vi "ROSTerminal.vi"() -> ()   [LabVIEW 2012]
doc: "Provides a space to debug any errors in code by:\n-allowing for testing connection to master\n-showing open nodes\n-linking to a website for viewing what is passed back and forth on a topic\n-linking to a website for the master to view what is passed back and forth\n-showing open logs\n-providing IP for you and Master"
uses:
  <userlib>/ROS for LabVIEW Software/ROS/Code/SubVIs/_ROSControl.ctl
  <userlib>/ROS for LabVIEW Software/ROS/Code/SubVIs/_ROSDirection.ctl
  <userlib>/ROS for LabVIEW Software/ROS/Code/_ROSDefinition.vi
  <vilib>/Platform/browser.llb/Open URL in Default Browser (string).vi
panel:
  in  "CloseServer":bool
  out "Queue Contents":string[](array[string])
  in  "ClearAllLogs":bool
  in  "CloseServers":bool
  in  "LabVIEW Servers":i32(listbox)
  in  "ClearOldLogs":bool
  in  "Web Logs":i32(listbox)
  in  "OpenNodes":bool
  in  "MasterWeb":bool
  in  "MyWeb":bool
  in  "UDP":bool
  out "My IP":string="http://192.168.1.8"
  in  "Done":bool
  out "Live":bool
  in  "Test":bool
  in  "Current Master":string="192.168.1.110:11311"
  # "Displays queue size and contents. Double click for\nmore information on a particular server."
  # "Show commands sent over TCP. \nDouble click to open a web page."
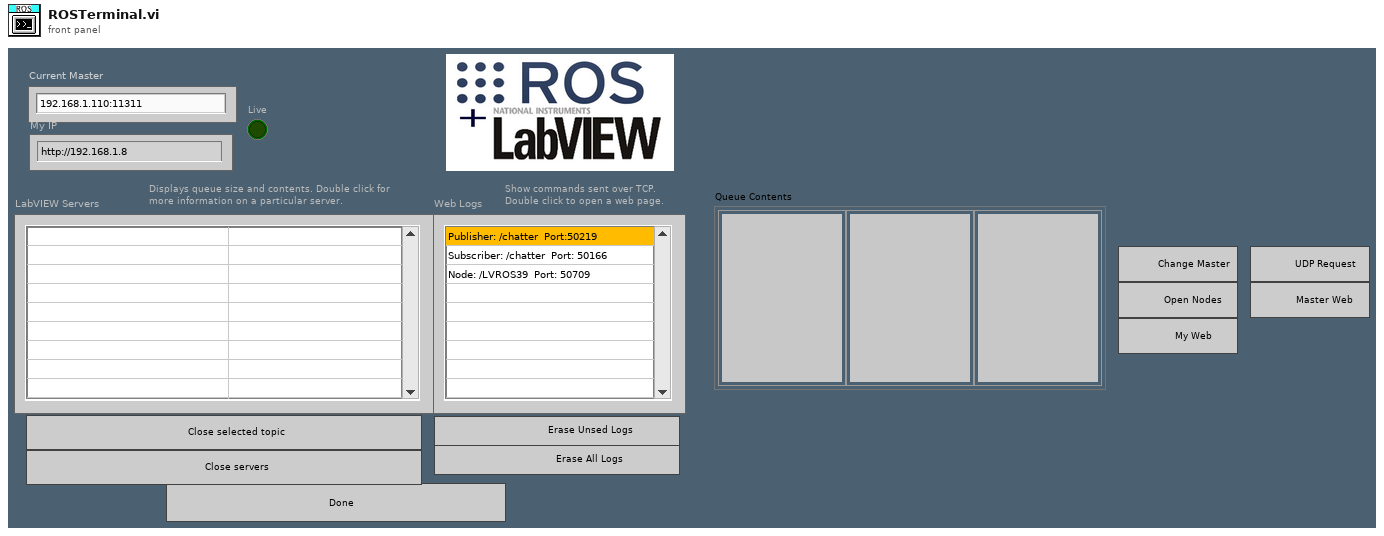
[diagram p1: front panel]
types:
  T1 = enum8{"Enabled", "Disabled", "Disabled and Grayed Out"}
  T2 = typedef "_ROSControl.ctl" = cluster{"topic port":u16, "Node":string, "topic":string, "type":string, "node port":u16, "error ":errorcluster, "Direction":T3, "Update (ms)":u16, "FIFO size":u16}
  T3 = typedef "_ROSDirection.ctl" = enum16{"Node", "Publisher", "Subscriber", "ServiceClient", "ServiceProvider"}
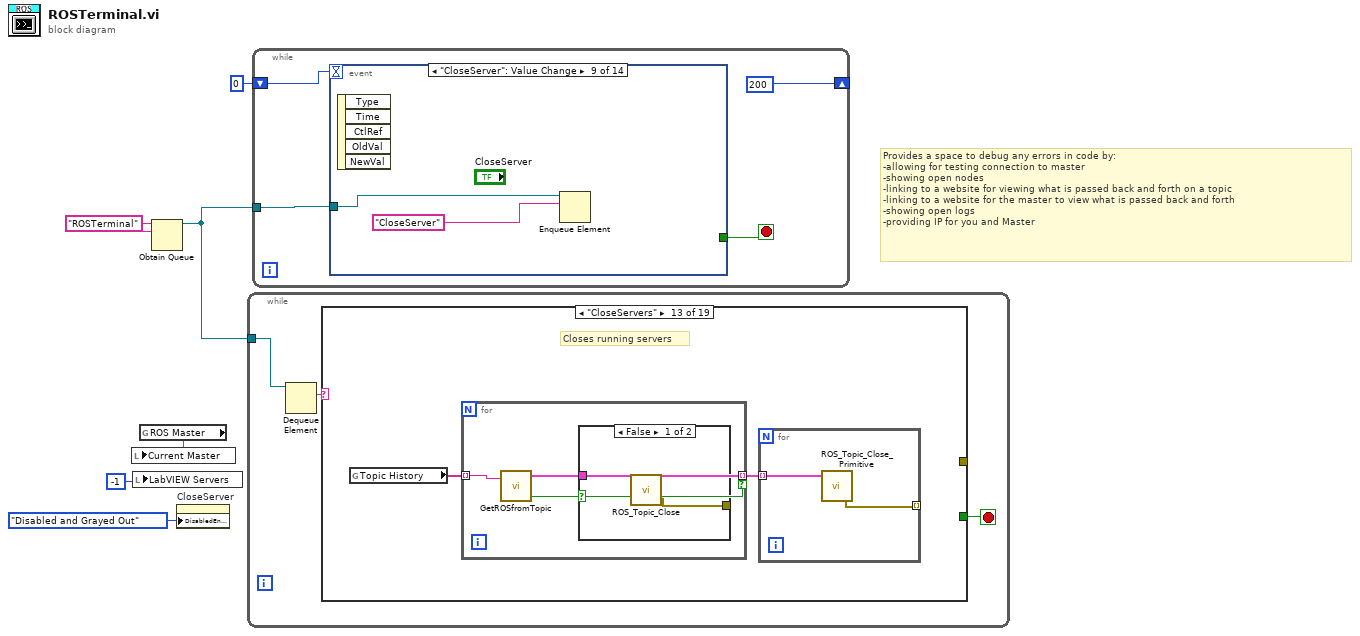
[diagram p0: block diagram]
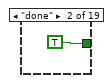
[diagram p3: hidden frame]
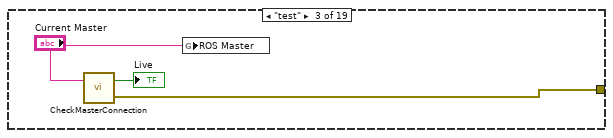
[diagram p4: hidden frame]
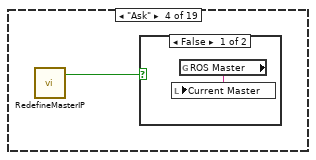
[diagram p5: hidden frame]
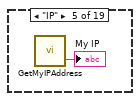
[diagram p7: hidden frame]
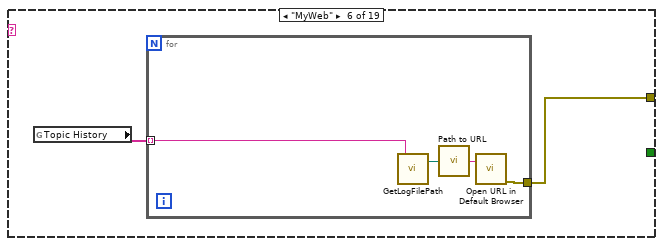
[diagram p8: hidden frame]
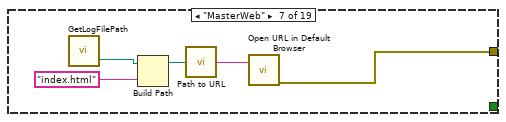
[diagram p9: hidden frame]
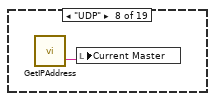
[diagram p10: hidden frame]
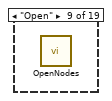
[diagram p11: hidden frame]
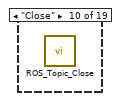
[diagram p12: hidden frame]
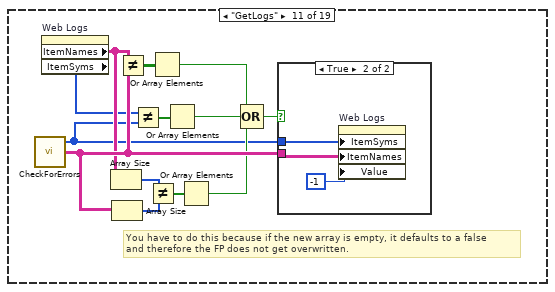
[diagram p13: hidden frame]
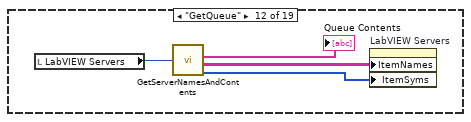
[diagram p15: hidden frame]
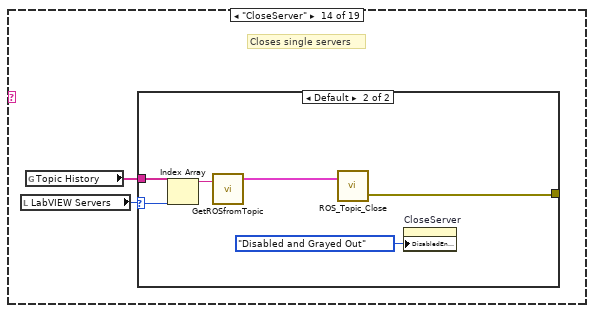
[diagram p17: hidden frame]
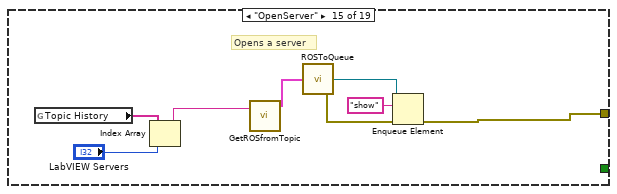
[diagram p19: hidden frame]
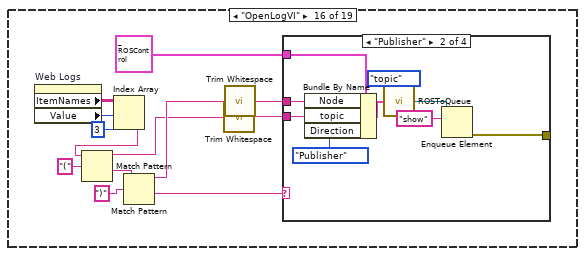
[diagram p20: hidden frame]
diagram:
  w5 = "ROSTerminal" ("name (unnamed)")
  # "Provides a space to debug any errors in code by:\n-allowing for testing connection to master\n-showing open nodes\n-linking to a website for viewing what is passed back and forth on a topic\n-linking to a website for the master to view what is passed back and forth\n-showing open logs\n-providing IP for you and Master"
  n1 = local write "LabVIEW Servers"(-1 ("Nodes")) -> ()
  n2 = global read "_ROSDefinition.vi" "ROS Master"() -> (w6:string)
  n3 = local write "Current Master"(w6) -> ()
  n4 = Obtain Queue(name (unnamed)=w5, element data type=w5) -> (queue out=w3:refnum<queue>)  [unwired: 3 in, 2 out]
  n5 = property on="CloseServer" class="Bool"("DisabledEnum"=T1."Disabled and Grayed Out" ("Disabled")) -> ()  [unwired: 2 in, 2 out]
  n6 = while {
    tunnel: w3 -> [w9]
    stop <- w7 stop-if-true
    n7 = Dequeue Element(queue=w9) -> (element=w8:string)  [unwired: 2 in, 3 out]
    n8 = case shown="\"CloseServers\"" w8 {
      tunnel: [_ TRUE _ _ _ _ _ _ _ _ _ _ _ _ _ _ _ _ _] -> w7
      tunnel: [_ _ w11 _ _ w18 w23 _ _ _ _ _ _ _ w67 _ _ _ _] -> _
      frame Default {
      }
      frame "done" {
      }
      frame "test" {
        n9 = call <userlib>:"CheckMasterConnection.vi"("Master IP"="Current Master") -> ("error out"=w11:errorcluster, "Master There?"=→"Live":bool)  [unwired: 1 in]
        n10 = global write "_ROSDefinition.vi" "ROS Master"("Current Master") -> ()
      }
      frame "Ask" {
        n11 = call <userlib>:"RedefineMasterIP.vi"() -> ("Abort?"=w14:bool)  [unwired: 2 in]
        n12 = case shown="False" w14 {
          frame False {
            n13 = global read "_ROSDefinition.vi" "ROS Master"() -> (w15:string)
            n14 = local write "Current Master"(w15) -> ()
          }
          frame True {
          }
        }
      }
      frame "IP" {
        n15 = call <userlib>:"GetMyIPAddress.vi"() -> ("URI"=→"My IP":string)  [unwired: 2 in, 1 out]
      }
      frame "MyWeb" {
        n16 = global read "_ROSDefinition.vi" "Topic History"() -> (w17:string[])
        n17 = for {
          tunnel: [w21] -> w18
          tunnel: w17 -> [w19] mode=indexing
          n18 = call <userlib>:"GetLogFilePath.vi"("Server name"=w19) -> ("LogPath"=w20:path)  [unwired: 1 in, 1 out]
          n19 = call <vilib>:"Path to URL.vi"("path"=w20) -> ("url"=w22:string)
          n20 = call-poly <vilib>:"Open URL in Default Browser.vi"("URL"=w22) -> ("error out"=w21:errorcluster)  [unwired: 5 in, 1 out]
        }
      }
      frame "MasterWeb" {
        n21 = call <userlib>:"GetLogFilePath.vi"() -> ("LogFolder"=w26:path)  [unwired: 2 in, 1 out]
        n22 = Build Path(base path=w26, name or relative path="index.html") -> (appended path=w24:path)
        n23 = call <vilib>:"Path to URL.vi"("path"=w24) -> ("url"=w27:string)
        n24 = call-poly <vilib>:"Open URL in Default Browser.vi"("URL"=w27) -> ("error out"=w23:errorcluster)  [unwired: 5 in, 1 out]
      }
      frame "UDP" {
        n25 = call <userlib>:"GetIPAddress.vi"() -> ("data out"=w28:string)  [unwired: 3 in]
        n26 = local write "Current Master"(w28) -> ()
      }
      frame "Open" {
        n27 = call <userlib>:"OpenNodes.vi"() -> ()  [unwired: 2 in]
      }
      frame "Close" {
        n28 = call <userlib>:"ROS_Topic_Close.vi"() -> ()  [unwired: 4 in, 1 out]
      }
      frame "GetLogs" {
        # "You have to do this because if the new array is empty, it defaults to a false\nand therefore the FP does not get overwritten."
        n29 = call <userlib>:"CheckForErrors.vi"() -> ("Symbols"=w30:i32[], "Logs"=w40:string[][])  [unwired: 2 in, 1 out]
        n30 = property on="Web Logs" class="MCListbox (strict)"() -> ("ItemNames"=w39:string[][], "ItemSyms"=w31:i32[])  [unwired: 2 in, 2 out]
        n31 = Array Size(array=w39) -> (size(s)=w38:i32[])
        n32 = Array Size(array=w40) -> (size(s)=w37:i32[])
        n33 = Not Equal?(x=w39, y=w40) -> (x != y?=w41:bool[][])
        n34 = Not Equal?(x=w31, y=w30) -> (x != y?=w32:bool[])
        n35 = Not Equal?(x=w38, y=w37) -> (x != y?=w36:bool[])
        n36 = Or Array Elements(Boolean array=w41) -> (logical OR=w35:bool)
        n37 = Or Array Elements(Boolean array=w32) -> (logical OR=w29:bool)
        n38 = Or Array Elements(Boolean array=w36) -> (logical OR=w34:bool)
        n39 = Compound Arithmetic op=OR(w35, w29, w34) -> (w33:bool)
        n40 = case shown="True" w33 {
          tunnel: w30 -> [_ w43]
          tunnel: w40 -> [_ w42]
          frame False {
          }
          frame True {
            n41 = property on="Web Logs" class="MCListbox (strict)"("ItemSyms"=w43, "ItemNames"=w42, "Value"=-1 ("Listbox")) -> ()  [unwired: 2 in, 2 out]
          }
        }
      }
      frame "GetQueue" {
        n42 = local read "LabVIEW Servers"() -> (w46:i32)
        n43 = call <userlib>:"GetServerNamesAndContents.vi"("Desired Server"=w46) -> ("Queue Contents"=→"Queue Contents":string[], "Nice Names"=w45:string[][], "Symbols"=w48:i32[])  [unwired: 1 out]
        n44 = property on="LabVIEW Servers" class="MCListbox (strict)"("ItemNames"=w45, "ItemSyms"=w48) -> ()  [unwired: 2 in, 2 out]
      }
      frame "CloseServers" {
        # "Closes running servers"
        n45 = global read "_ROSDefinition.vi" "Topic History"() -> (w50:string[])
        n46 = for {
          tunnel: w50 -> [w55] mode=indexing
          tunnel: [w54] -> w49 mode=indexing if=w53
          n47 = call <userlib>:"GetROSfromTopic.vi"("Topic"=w55) -> ("ROS"=w54:T2, "Node?"=w53:bool)  [unwired: 1 in, 1 out]
          n48 = case shown="False" w53 {
            tunnel: w54 -> [w57 _]
            tunnel: [w56 _] -> _
            frame False {
              n49 = call <userlib>:"ROS_Topic_Close.vi"("ROS in"=w57) -> ("error out"=w56:errorcluster)  [unwired: 3 in]
            }
            frame True {
            }
          }
        }
        n50 = for {
          tunnel: w49 -> [w52] mode=indexing
          tunnel: [w51] -> _ mode=indexing
          n51 = call <userlib>:"ROS_Topic_Close_Primitive.vi"("ROS in"=w52) -> ("error out"=w51:errorcluster)  [unwired: 2 in]
        }
      }
      frame "CloseServer" {
        # "Closes single servers"
        n52 = local read "LabVIEW Servers"() -> (w58:i32)
        n53 = global read "_ROSDefinition.vi" "Topic History"() -> (w59:string[])
        n54 = case shown="Default" w58 {
          selector: w58 -> [_ w64]
          tunnel: w59 -> [_ w63]
          tunnel: [_ w60] -> _
          frame -1 {
          }
          frame Default {
            n55 = Index Array(array=w63, index=w64) -> (element=w62:string)
            n56 = call <userlib>:"GetROSfromTopic.vi"("Topic"=w62) -> ("ROS"=w65:T2)  [unwired: 1 in, 2 out]
            n57 = call <userlib>:"ROS_Topic_Close.vi"("ROS in"=w65) -> ("error out"=w60:errorcluster)  [unwired: 3 in]
            n58 = property on="CloseServer" class="Bool"("DisabledEnum"=T1."Disabled and Grayed Out" ("Disabled")) -> ()  [unwired: 2 in, 2 out]
          }
        }
      }
      frame "OpenServer" {
        # "Opens a server"
        n59 = global read "_ROSDefinition.vi" "Topic History"() -> (w72:string[])
        n60 = Index Array(array=w72, index="LabVIEW Servers") -> (element=w70:string)
        n61 = call <userlib>:"GetROSfromTopic.vi"("Topic"=w70) -> ("ROS"=w68:T2)  [unwired: 1 in, 2 out]
        n62 = call <userlib>:"ROSToQueue.vi"("ROS"=w68) -> ("error out"=w66:errorcluster, "queue"=w69:refnum<queue>)  [unwired: 3 in]
        n63 = Enqueue Element(queue=w69, element="show", error in (no error)=w66) -> (error out=w67:errorcluster)  [unwired: 1 in, 2 out]
      }
      frame "OpenLogVI" {
        n64 = property on="Web Logs" class="MCListbox (strict)"() -> ("ItemNames"=w78:string[][], "Value"=w79:i32)  [unwired: 2 in, 2 out]
        n65 = Index Array(array=w78, index (row)=w79, index (col)=3 ("disabled index (col)")) -> (element=w83:string)
        n66 = Match Pattern(string=w83, regular expression="(") -> (before substring=w75:string, after substring=w84:string)  [unwired: 1 in, 2 out]
        n67 = Match Pattern(string=w84, regular expression=")") -> (before substring=w77:string, after substring=w86:string)  [unwired: 1 in, 2 out]
        n68 = call <vilib>:"Trim Whitespace.vi"("string"=w75) -> ("trimmed string"=w74:string)  [unwired: 1 in]
        n69 = call <vilib>:"Trim Whitespace.vi"("string"=w77) -> ("trimmed string"=w76:string)  [unwired: 1 in]
        n70 = case shown="\"Publisher\"" w86 {
          tunnel: T2 {"topic port"=0, "Node"="/fred", "topic"="/robot/head/command_head_nod", "type"="std_msgs/Bool", "node port"=59377, "error "={"status"=FALSE, "code"=0, "source"=""}, "Direction"=enum."Publisher", "Update (ms)"=1, "FIFO size"=1} ("ROS") -> [_ w95 w104 w113]
          tunnel: w74 -> [_ w89 w99 w108]
          tunnel: w76 -> [_ w88 w98 w107]
          tunnel: [_ w87 w96 w105] -> _
          frame Default {
          }
          frame "Publisher" {
            n71 = Bundle By Name(cluster=w95, "Node"=w88, "topic"=w89, "Direction"=_ROSDirection."Publisher") -> (w94:T2)
            n72 = call <userlib>:"ROSToQueue.vi"("ROS"=w94, "Name"=enum16{"topic", "node"}."topic") -> ("queue"=w92:refnum<queue>)  [unwired: 2 in, 1 out]
            n73 = Enqueue Element(queue=w92, element="show") -> (error out=w87:errorcluster)  [unwired: 2 in, 2 out]
          }
          frame "Subscriber" {
            n74 = Bundle By Name(cluster=w104, "Node"=w98, "topic"=w99, "Direction"=_ROSDirection."Subscriber") -> (w103:T2)
            n75 = call <userlib>:"ROSToQueue.vi"("ROS"=w103, "Name"=enum16{"topic", "node"}."topic") -> ("queue"=w101:refnum<queue>)  [unwired: 2 in, 1 out]
            n76 = Enqueue Element(queue=w101, element="show") -> (error out=w96:errorcluster)  [unwired: 2 in, 2 out]
          }
          frame "Node" {
            n77 = Bundle By Name(cluster=w113, "Node"=w107, "topic"=w108, "Direction"=_ROSDirection."Node") -> (w112:T2)
            n78 = call <userlib>:"ROSToQueue.vi"("ROS"=w112, "Name"=enum16{"topic", "node"}."node") -> ("queue"=w110:refnum<queue>)  [unwired: 2 in, 1 out]
            n79 = Enqueue Element(queue=w110, element="show") -> (error out=w105:errorcluster)  [unwired: 2 in, 2 out]
          }
        }
      }
      frame "OpenLogs" {
        n80 = property on="Web Logs" class="MCListbox (strict)"() -> ("ItemNames"=w118:string[][])  [unwired: 2 in, 2 out]
        n81 = Index Array(array=w118, index (row)="Web Logs") -> (element=w117:string[])  [unwired: 1 in]
        n82 = Index Array(array=w117, index=1) -> (element=w114:string)
        n83 = call-poly <vilib>:"Open URL in Default Browser.vi"("URL"=w114) -> ()  [unwired: 5 in, 2 out]
      }
      frame "EraseLogs" {
        n84 = call <userlib>:"CheckForErrors.vi"() -> ("Symbols"=w120:i32[], "Paths"=w119:path[])  [unwired: 2 in, 1 out]
        n85 = for {
          tunnel: w120 -> [w122] mode=indexing
          tunnel: w119 -> [w121] mode=indexing
          n86 = case shown="0" w122 {
            tunnel: [w124 _] -> _
            tunnel: w121 -> [w123 _]
            frame 0 {
              n87 = Delete(path (use dialog)=w123) -> (error out=w124:errorcluster)  [unwired: 4 in, 2 out]
            }
            frame Default {
            }
          }
        }
      }
      frame "EraseAll" {
        n88 = call <userlib>:"CheckForErrors.vi"() -> ("Paths"=w125:path[])  [unwired: 2 in, 2 out]
        n89 = for {
          tunnel: w125 -> [w127] mode=indexing
          tunnel: [w126] -> _ mode=indexing
          n90 = Delete(path (use dialog)=w127) -> (error out=w126:errorcluster)  [unwired: 4 in, 2 out]
        }
      }
    }
  }
  n91 = while {
    tunnel: w3 -> [w131]
    shift-right: [200 ("timeout in ms (-1)")] -> _
    shift-left: 0 ("timeout in ms (-1)") -> [w128]
    stop <- w130 stop-if-true
    n92 = event shown="[8] \"CloseServer\": Value Change" {
      selector: _ -> [_ _ _ _ _ _ _ _ _ _ _ _ _ _]
      dyn-events: _ -> [_ _ _ _ _ _ _ _ _ _ _ _ _ _]
      timeout: w128 -> [_ _ _ _ _ _ _ _ _ _ _ _ _ _]
      tunnel: w131 -> [w133 w141 w143 w145 w147 _ w150 w152 w154 w158 w162 w164 w166 w169]
      tunnel: [_ _ _ _ _ _ _ _ _ _ _ _ _ "Done"] -> w130
      event Timeout {
        n93 = event-data() -> ()  [unwired: 1 in, 1 out]
        n94 = Get Queue Status(queue=w133) -> (# elements in queue=w132:i32)  [unwired: 2 in, 7 out]
        n95 = case shown="0" w132 {
          tunnel: string[] ["IP", "GetLogs", "test", "GetQueue"] -> [_ w136]
          tunnel: w133 -> [_ w135]
          frame Default {
          }
          frame 0 {
            n96 = for {
              shift-right: [w139] -> _
              shift-left: w135 -> [w138]
              tunnel: w136 -> [w137] mode=indexing
              n97 = Enqueue Element(queue=w138, element=w137) -> (queue out=w139:refnum<queue>)  [unwired: 2 in, 2 out]
            }
          }
        }
      }
      event "Test", "Current Master": Value Change {
        n98 = event-data() -> ()  [unwired: 1 in, 1 out]
        n99 = Enqueue Element(queue=w141, element="Ask") -> ()  [unwired: 2 in, 3 out]
      }
      event "MyWeb": Value Change {
        n100 = event-data() -> ()  [unwired: 1 in, 1 out]
        n101 = Enqueue Element(queue=w143, element="MyWeb") -> ()  [unwired: 2 in, 3 out]
      }
      event "UDP": Value Change {
        n102 = event-data() -> ()  [unwired: 1 in, 1 out]
        n103 = Enqueue Element(queue=w145, element="UDP") -> ()  [unwired: 2 in, 3 out]
      }
      event "LabVIEW Servers": Double Click {
        n104 = event-data() -> ()  [unwired: 1 in, 1 out]
        n105 = Enqueue Element(queue=w147, element="OpenServer") -> ()  [unwired: 2 in, 3 out]
      }
      event "LabVIEW Servers": Mouse Up {
        n106 = event-data() -> ()  [unwired: 1 in, 1 out]
        n107 = property on="CloseServer" class="Bool"("DisabledEnum"=T1."Enabled" ("Disabled")) -> ()  [unwired: 2 in, 2 out]
      }
      event "Web Logs": Double Click {
        n108 = event-data() -> ()  [unwired: 1 in, 1 out]
        n109 = Enqueue Element(queue=w150, element="OpenLogs") -> ()  [unwired: 2 in, 3 out]
      }
      event "CloseServers": Value Change {
        n110 = event-data() -> ()  [unwired: 1 in, 5 out]
        n111 = Enqueue Element(queue=w152, element="CloseServers") -> ()  [unwired: 2 in, 3 out]
      }
      event "CloseServer": Value Change {
        n112 = event-data() -> ()  [unwired: 1 in, 5 out]
        n113 = Enqueue Element(queue=w154, element="CloseServer") -> ()  [unwired: 2 in, 3 out]
      }
      event "ClearOldLogs": Value Change {
        n114 = event-data() -> ()  [unwired: 1 in, 5 out]
        n115 = Enqueue Element(queue=w158, element="EraseLogs") -> (queue out=w156:refnum<queue>)  [unwired: 2 in, 2 out]
        n116 = Enqueue Element(queue=w156, element="GetLogs") -> ()  [unwired: 2 in, 3 out]
      }
      event "ClearAllLogs": Value Change {
        n117 = event-data() -> ()  [unwired: 1 in, 5 out]
        n118 = Enqueue Element(queue=w162, element="EraseAll") -> (queue out=w160:refnum<queue>)  [unwired: 2 in, 2 out]
        n119 = Enqueue Element(queue=w160, element="GetLogs") -> ()  [unwired: 2 in, 3 out]
      }
      event "OpenNodes": Value Change {
        n120 = event-data() -> ()  [unwired: 1 in, 1 out]
        n121 = Enqueue Element(queue=w164, element="Open") -> ()  [unwired: 2 in, 3 out]
      }
      event "MasterWeb": Value Change {
        n122 = event-data() -> ()  [unwired: 1 in, 1 out]
        n123 = Enqueue Element(queue=w166, element="MasterWeb") -> ()  [unwired: 2 in, 3 out]
      }
      event "Done": Value Change {
        n124 = event-data() -> ()  [unwired: 1 in, 1 out]
        n125 = Enqueue Element(queue=w169, element="done") -> ()  [unwired: 2 in, 3 out]
      }
    }
  }
